vi "Pre Launch Init.vi"(11 "ConfigurableActor in":refnum<class "ConfigurableActor.lvclass">) -> (0 "error out":errorcluster, 3 "ConfigurableActor out":refnum<class "ConfigurableActor.lvclass">)   [LabVIEW 2014, in "ConfigurableActor.lvclass"]
doc: "(<B>Filename</B>: Actor Framework.lvlib:Actor.lvclass:Pre Launch Init.vi)\n\nDefines behavior that occurs after the Launch Nested Actor method is invoked but before the actor's Actor Core method begins running.\n\nBy default, this method does nothing. A descendant class may override it to define behavior."
uses:
  ConfigurableActor.lvclass
  ConfigurableActor.lvclass/ConfigurableActor.ctl
  <vilib>/LabVIEW Open Source/Configuration Manager/Manager/ConfigManager.lvclass
  <vilib>/ActorFramework/Actor/Actor.lvclass
  <vilib>/LabVIEW Open Source/Configuration Manager/Cache/ConfigManager.Cache.lvclass
  <vilib>/LabVIEW Open Source Project/Unicity/UniqueName/Registry/NameRegistry.lvclass
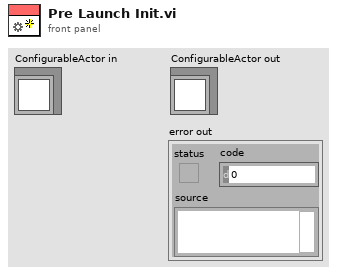
[diagram p1: front panel]
types:
  T1 = typedef "UniqueName.lvlib/NameRegistry.lvclass/RegistryConfiguration.ctl" = cluster{"Delimiter":refnum<class "Delimiter.lvclass">, "RandomStringGenerator":refnum<class "RandomStringGenerator.lvclass">, "UniquenessCriteria":refnum<class "UniquenessCriteria.lvclass">, "StringIncrement":refnum<class "StringIncrement.lvclass">}
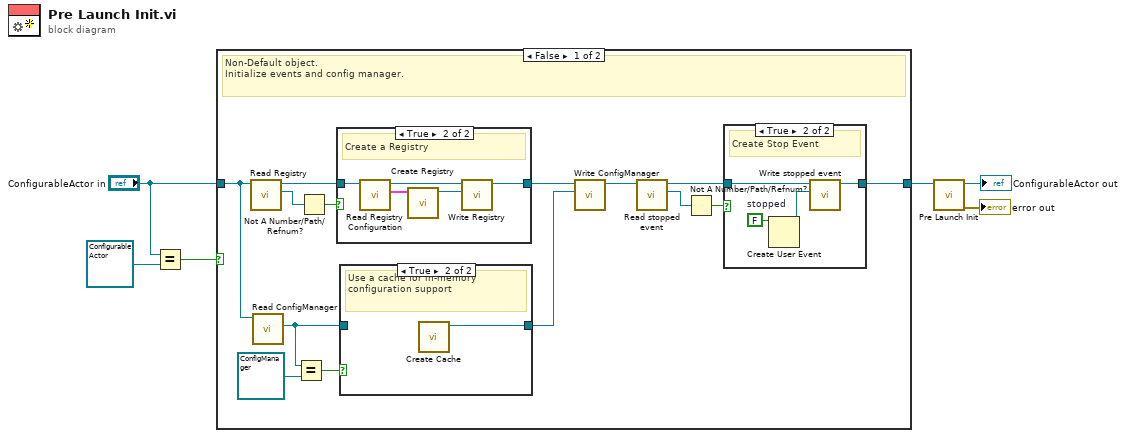
[diagram p0: block diagram]
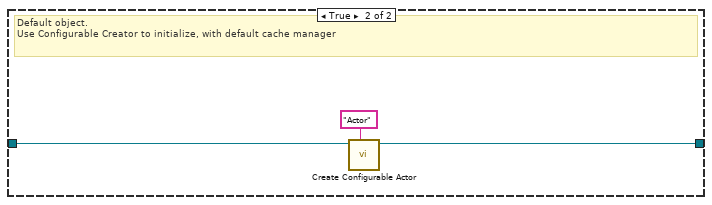
[diagram p5: hidden frame]
diagram:
  n1 = Equal?(x="ConfigurableActor in", y=refnum<class "ConfigurableActor.lvclass"> refnum ("ConfigurableActor in")) -> (x = y?=w3:bool)
  n2 = case shown="False" w3 {
    tunnel: "ConfigurableActor in" -> [w8 w34]
    tunnel: [w20 w36] -> w1
    frame False {
      # "Non-Default object.\nInitialize events and config manager."
      n3 = call "Read Registry.vi"("ConfigurableActor in"=w8) -> ("Registry"=w9:refnum<data-value>, "ConfigurableActor out"=w11:refnum<class "ConfigurableActor.lvclass">)  [unwired: 9 in]
      n4 = call "Read ConfigManager.vi"("ConfigurableActor in"=w8) -> ("ConfigManager"=w16:refnum<class "ConfigManager.lvclass">)  [unwired: 8 in, 2 out]
      n5 = Equal?(x=w16, y=refnum<class "ConfigManager.lvclass"> refnum) -> (x = y?=w17:bool)
      n6 = Not A Number/Path/Refnum?(number/path/refnum=w9) -> (NaN/Path/Refnum?=w10:bool)
      n7 = case shown="True" w10 {
        tunnel: w11 -> [w21 w24]
        tunnel: [w21 w26] -> w7
        frame False {
          # "Registry already created"
        }
        frame True {
          # "Create a Registry"
          n8 = call "Read Registry Configuration.vi"("ConfigurableActor in"=w24) -> ("Registry Configuration"=w22:T1, "ConfigurableActor out"=w23:refnum<class "ConfigurableActor.lvclass">)  [unwired: 9 in]
          n9 = call <vilib>:"Create Registry.vi"("Registry Configuration"=w22) -> ("Registry"=w25:refnum<data-value>)  [unwired: 9 in, 1 out]
          n10 = call "Write Registry.vi"("Registry"=w25, "ConfigurableActor in"=w23) -> ("ConfigurableActor out"=w26:refnum<class "ConfigurableActor.lvclass">)  [unwired: 9 in]
        }
      }
      n11 = case shown="True" w17 {
        tunnel: [w32 w33] -> w19
        tunnel: w16 -> [w32 _]
        frame False {
        }
        frame True {
          # "Use a cache for in-memory\nconfiguration support"
          n12 = call <vilib>:"Create Cache.vi"() -> ("ConfigManager.Cache"=w33:refnum<class "ConfigManager.Cache.lvclass">)  [unwired: 11 in]
        }
      }
      n13 = call "Write ConfigManager.vi"("ConfigManager"=w19, "ConfigurableActor in"=w7) -> ("ConfigurableActor out"=w15:refnum<class "ConfigurableActor.lvclass">)  [unwired: 8 in, 1 out]
      n14 = call "Read stopped event.vi"("ConfigurableActor in"=w15) -> ("stopped event"=w13:refnum<user-event>, "ConfigurableActor out"=w14:refnum<class "ConfigurableActor.lvclass">)  [unwired: 8 in, 1 out]
      n15 = Not A Number/Path/Refnum?(number/path/refnum=w13) -> (NaN/Path/Refnum?=w12:bool)
      n16 = case shown="True" w12 {
        tunnel: [w27 w29] -> w20
        tunnel: w14 -> [w27 w30]
        frame False {
        }
        frame True {
          w31 = FALSE  # stopped
          # "Create Stop Event"
          n17 = Create User Event(user event datatype=w31) -> (user event=w28:refnum<user-event>)  [unwired: 1 in, 1 out]
          n18 = call "Write stopped event.vi"("stopped event"=w28, "ConfigurableActor in"=w30) -> ("ConfigurableActor out"=w29:refnum<class "ConfigurableActor.lvclass">)  [unwired: 8 in, 1 out]
        }
      }
    }
    frame True {
      # "Default object. \nUse Configurable Creator to initialize, with default cache manager"
      n19 = call "Create Configurable Actor.vi"("Name"="Actor", "ConfigurableActor"=w34) -> ("ConfigurableActor out"=w36:refnum<class "ConfigurableActor.lvclass">)  [unwired: 8 in, 1 out]
    }
  }
  n20 = call-parent "Pre Launch Init.vi"("Actor in"=w1) -> ("error out"=→"error out":errorcluster, "Actor out"=→"ConfigurableActor out":refnum<class "ConfigurableActor.lvclass">)  [unwired: 9 in]
